vi "Set Handshake.vi"(8 "error in (no error)":errorcluster, 11 "Panel in":refnum<class "Station Actor.lvclass">) -> (0 "error out":errorcluster, 3 "Panel out":refnum<class "Station Actor.lvclass">)   [LabVIEW 2019, in "Station Actor.lvlib" / "Station Actor.lvclass"]
uses:
  Station Actor.lvclass
  Station Actor.lvclass/Station Actor.ctl
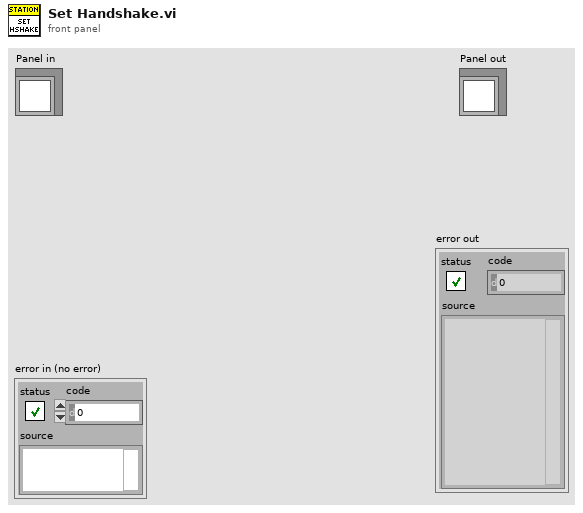
[diagram p1: front panel]
types:
  T1 = typedef "Panel.lvlib/Panel.lvclass/Tester Tx Dataset.ctl" = cluster{"Fault":bool, "StepNo":u32, "Ready":bool, "HighVoltage":bool, "TestRunning":bool, "ResultsReady":bool, "Results":u32, "ElapsedTime":u32, "Online":bool, "TimeCompleted":i32[], "Timeout":bool, "Heartbeat":bool}
  T2 = typedef "Panel.lvlib/Panel.lvclass/Tester Rx Dataset.ctl" = cluster{"Start":bool, "NestStatus":bool, "PalletID":u32, "BarcodeData":string, "StepEcho":u32, "Cylinder_1":bool, "Cylinder_2":bool, "Cylinder_3":bool, "Cylinder_4":bool, "Cylinder_5":bool, "ResultsAck":bool, "Reset":bool, "Stop":bool, "FaultCode":u32}
  T3 = typedef "Station Actor.lvlib/Station Actor.lvclass/Tester Rx Dataset.ctl" = cluster{"Start":bool, "NestStatus":bool, "PalletID":u32, "BarcodeData":string, "StepEcho":u32, "Cylinder_1":bool, "Cylinder_2":bool, "Cylinder_3":bool, "Cylinder_4":bool, "Cylinder_5":bool, "ResultsAck":bool, "Reset":bool, "Stop":bool, "FaultCode":u32}
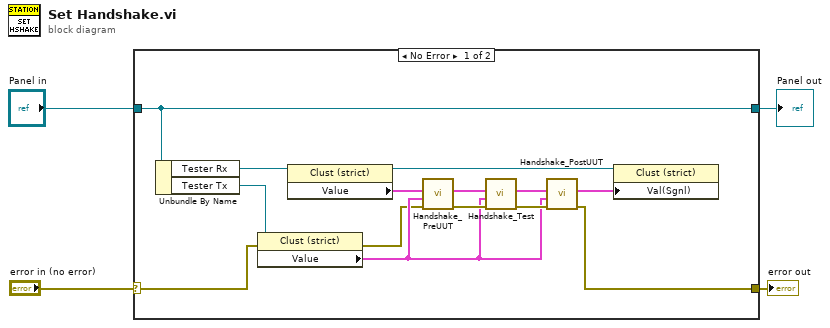
[diagram p0: block diagram]
diagram:
  n1 = case shown="No Error" "error in (no error)" {
    selector: "error in (no error)" -> [w5 w20]
    tunnel: [w7 w20] -> w3
    tunnel: [w18 w19] -> w1
    tunnel: "Panel in" -> [w18 w19]
    frame No Error {
      n2 = Unbundle By Name(w18) -> ("Tester Rx"=w17:refnum<vi>, "Tester Tx"=w16:refnum<vi>)
      n3 = property class="Clust (strict)"(reference=w16, error in=w5) -> (error out=w6:errorcluster, "Value"=w9:T1)  [unwired: 1 out]
      n4 = property class="Clust (strict)"(reference=w17) -> (reference out=w15:refnum<vi>, "Value"=w12:T2)  [unwired: 1 in, 1 out]
      n5 = call "Handshake_PreUUT.vi"("error in"=w6, "Tester Tx"=w9, "Tester Rx In"=w12) -> ("error out"=w14:errorcluster, "Tester Rx out"=w11:T3)  [unwired: 7 in]
      n6 = call "Handshake_Test.vi"("error in"=w14, "Tester Tx"=w9, "Tester Rx In"=w11) -> ("error out"=w13:errorcluster, "Tester Rx out"=w10:T3)  [unwired: 7 in]
      n7 = call "Handshake_PostUUT.vi"("error in"=w13, "Tester Tx"=w9, "Tester Rx In"=w10) -> ("error out"=w7:errorcluster, "Tester Rx out"=w8:T3)  [unwired: 7 in]
      n8 = property class="Clust (strict)"(reference=w15, "Val(Sgnl)"=w8) -> ()  [unwired: 1 in, 2 out]
    }
    frame Error {
    }
  }
  "error out" <- w3
  "Panel out" <- w1
